vi "默认配置对话框.vi"() -> (2 "check？":bool, 3 "默认配置选择输出":T1)   [LabVIEW 2016]
uses:
  <vilib>/Utility/miscctls.llb/LVPointTypeDef.ctl
panel:
  in  "取消":bool
  in  "确认":bool
  in  "默认配置选择":T1
  # "请选择默认配置表"
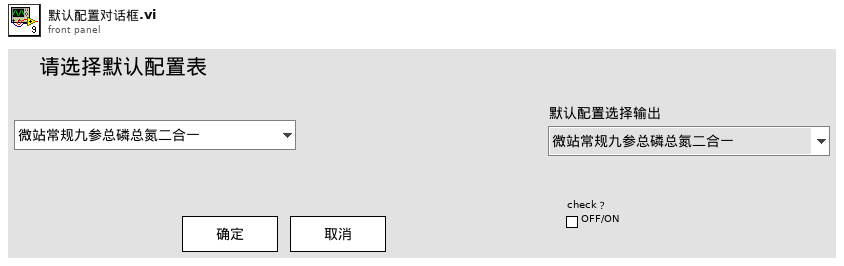
[diagram p1: front panel]
types:
  T1 = typedef "配置表选择.ctl" = enum16{"微站常规九参总磷总氮二合一", "微站常规八参氨氮总磷二合一", "微站常规九参", "微站常规八参", "固定站常规九参", "浮船常规九参总磷总氮二合一", "浮船常规九参"}
  T2 = typedef "LVPointTypeDef.ctl" = cluster{"Horizontal":i16, "Vertical":i16}
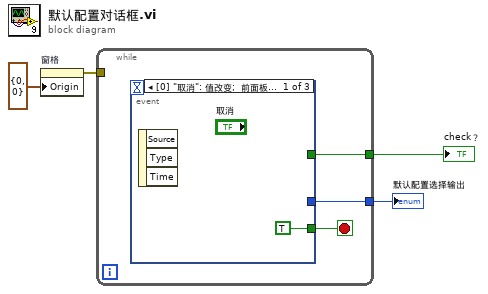
[diagram p0: block diagram]
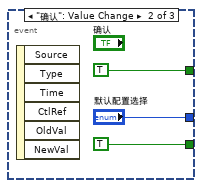
[diagram p2: hidden frame]
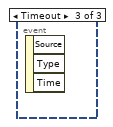
[diagram p3: hidden frame]
diagram:
  n1 = property on="窗格" class="Pane"("Origin"=T2 {"Horizontal"=0, "Vertical"=0} ("原点")) -> (error out=w1:errorcluster)  [unwired: 2 in, 1 out]
  n2 = while {
    tunnel: [w7] -> w4
    tunnel: [w5] -> w3
    tunnel: w1 -> [_]
    stop <- w6 stop-if-true
    n3 = event shown="[0] \"取消\": 值改变;  前面板关闭" {
      selector: _ -> [_ _ _]
      dyn-events: _ -> [_ _ _]
      timeout: _ -> [_ _ _]
      tunnel: [_ "默认配置选择" _] -> w7
      tunnel: [TRUE TRUE _] -> w6
      tunnel: [_ TRUE _] -> w5
      event "取消": Value Change; Panel Close {
        n4 = event-data() -> ()  [unwired: 1 in, 3 out]
      }
      event "确认": Value Change {
        n5 = event-data() -> ()  [unwired: 1 in, 6 out]
      }
      event Timeout {
        n6 = event-data() -> ()  [unwired: 1 in, 3 out]
      }
    }
  }
  "check？" <- w3
  "默认配置选择输出" <- w4
